vi "Load BIN File Information.vi"(8 "error in (no error)":errorcluster, 11 "File Path":path) -> (0 "error out":errorcluster, 1 "BIN dataset Information":T1, 2 "offset (in bytes)":i64, 3 "File Path out":path, 4 "CPU (s)":dbl, 5 "Data Description":string)   [LabVIEW 2021, in "PicoQuant.lvlib"]
uses:
  BIN File Information.ctl
  PicoQuant.lvlib
  Time/Time.lvlib
  Variant/Variant.lvlib
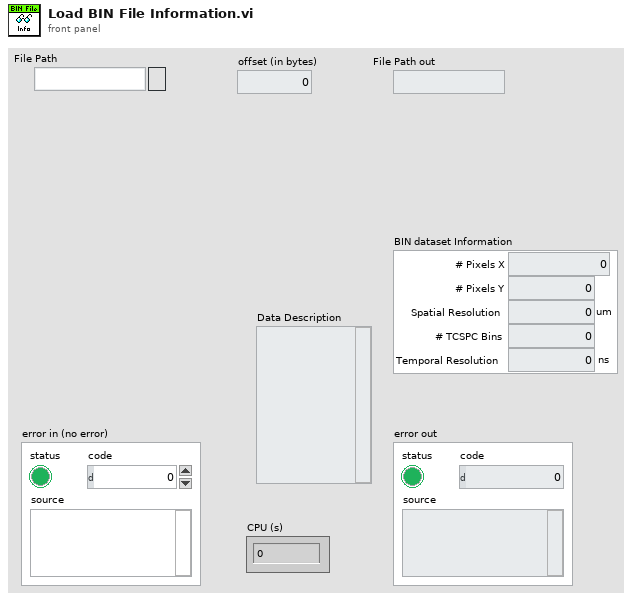
[diagram p1: front panel]
types:
  T1 = typedef "PicoQuant.lvlib/BIN File Information.ctl" = cluster{"# Pixels X":i32, "# Pixels Y":i32, "Spatial Resolution":dbl[unit], "# TCSPC Bins":i32, "Temporal Resolution":dbl[unit]}
  T2 = enum16{"open", "replace", "create", "open or create", "replace or create", "replace or create with confirmation"}
  T3 = enum16{"big-endian, network order", "native, host order", "little-endian"}
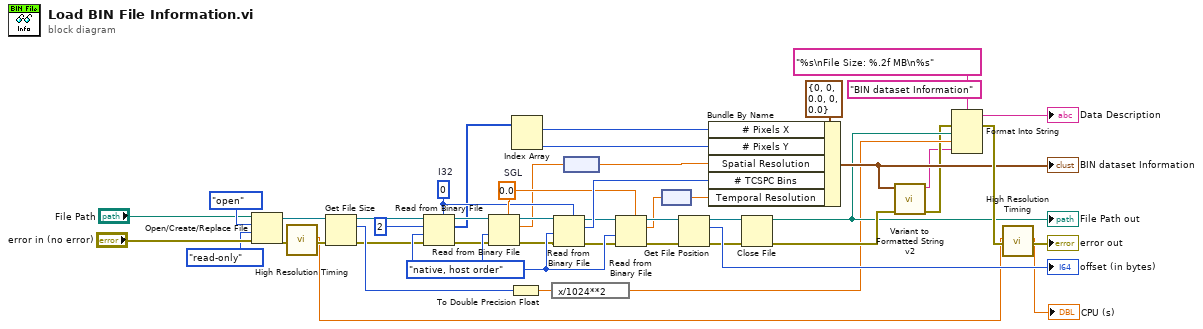
[diagram p0: block diagram]
diagram:
  (unwired) "BIN dataset Information" ("Label")
  w23 = sgl 0.0  # SGL
  w33 = T3."native, host order" ("byte order (0:big-endian, network order)")
  w20 = 0  # I32
  n1 = Open/Create/Replace File(file path (use dialog)="File Path", error in="error in (no error)", operation (0:open)=T2."open", access (0:read/write)=enum16{"read/write", "read-only", "write-only"}."read-only") -> (refnum out=w6:refnum<file>, error out=w9:errorcluster)  [unwired: 2 in, 1 out]
  n2 = call "High Resolution Timing.vi"("Error In"=w9) -> ("elapsed (relative) seconds"=w2:dbl, "Error Out"=w4:errorcluster)  [unwired: 16 in, 1 out]
  n3 = Get File Size(file=w6, error in=w4) -> (refnum out=w26:refnum<file>, size (in bytes)=w28:i64, 0:w27:errorcluster)
  n4 = Read from Binary File(5:w20, 8:w27, 9:w33, 10:2 ("count (1)"), 11:w26) -> (0:w14:errorcluster, 2:w13:i32[], 3:w15:refnum<file>)  [unwired: 1 in, 1 out]
  n5 = Read from Binary File(5:w23, 8:w14, 9:w33, 11:w15) -> (0:w19:errorcluster, 2:w16:sgl, 3:w18:refnum<file>)  [unwired: 2 in, 1 out]
  n6 = To Double Precision Float(number=w28) -> (double precision float=w29:dbl)
  n7 = Index Array(array=w13) -> (element #1=w35:i32, element #2=w36:i32)  [unwired: 2 in]
  n8 = expression code="x/1024**2"(w29) -> (w39:dbl)
  n9 = Read from Binary File(5:w20, 8:w19, 9:w33, 11:w18) -> (0:w21:errorcluster, 2:w37:i32, 3:w22:refnum<file>)  [unwired: 2 in, 1 out]
  n10 = node(w16) -> (w17:sgl[unit])
  n11 = Read from Binary File(5:w23, 8:w21, 9:w33, 11:w22) -> (0:w32:errorcluster, 2:w24:sgl, 3:w43:refnum<file>)  [unwired: 2 in, 1 out]
  n12 = node(w24) -> (w25:sgl[unit])
  n13 = Get File Position(4:w32, 7:w43) -> (0:w42:errorcluster, 2:→"offset (in bytes)":i64, 3:w44:refnum<file>)
  n14 = Bundle By Name(cluster=T1 {"# Pixels X"=0, "# Pixels Y"=0, "Spatial Resolution"=0.0, "# TCSPC Bins"=0, "Temporal Resolution"=0.0} ("BIN dataset Information"), "# Pixels X"=w35, "# Pixels Y"=w36, "Spatial Resolution"=w17, "# TCSPC Bins"=w37, "Temporal Resolution"=w25) -> (w41:T1)
  "BIN dataset Information" <- w41
  n15 = Close File(refnum=w44, error in=w42) -> (path=w40:path, error out=w46:errorcluster)
  "File Path out" <- w40
  n16 = call "Variant to Formatted String v2.vi"("error in (no error)"=w46, "Anything"=w41) -> ("error out"=w34:errorcluster, "String"=w30:string)  [unwired: 8 in]
  n17 = Format Into String(format string="%s\nFile Size: %.2f MB\n%s", error in=w34, w40, w39, w30) -> (resulting string=→"Data Description":string, error out=w47:errorcluster)  [unwired: 1 in]
  n18 = call "High Resolution Timing.vi"("relative seconds (NaN)"=w2, "Error In"=w47) -> ("elapsed (relative) seconds"=→"CPU (s)":dbl, "Error Out"=→"error out":errorcluster)  [unwired: 15 in, 1 out]
